vi "CreateNewFile.vi"(8 "error in (no error)":errorcluster, 11 "BenchParent in":refnum<class "BenchParent.lvclass">) -> (0 "error out":errorcluster, 2 "file path out":path, 3 "BenchParent out":refnum<class "BenchParent.lvclass">)   [LabVIEW 2024, in "BenchParent.lvclass"]
uses:
  BenchParent.lvclass
  <vilib>/numeric/Random Number (Range) DBL.vi
  BenchParent.lvclass/BenchParent.ctl
panel:
  out "Waveform Graph":waveform(dbl)(graph)
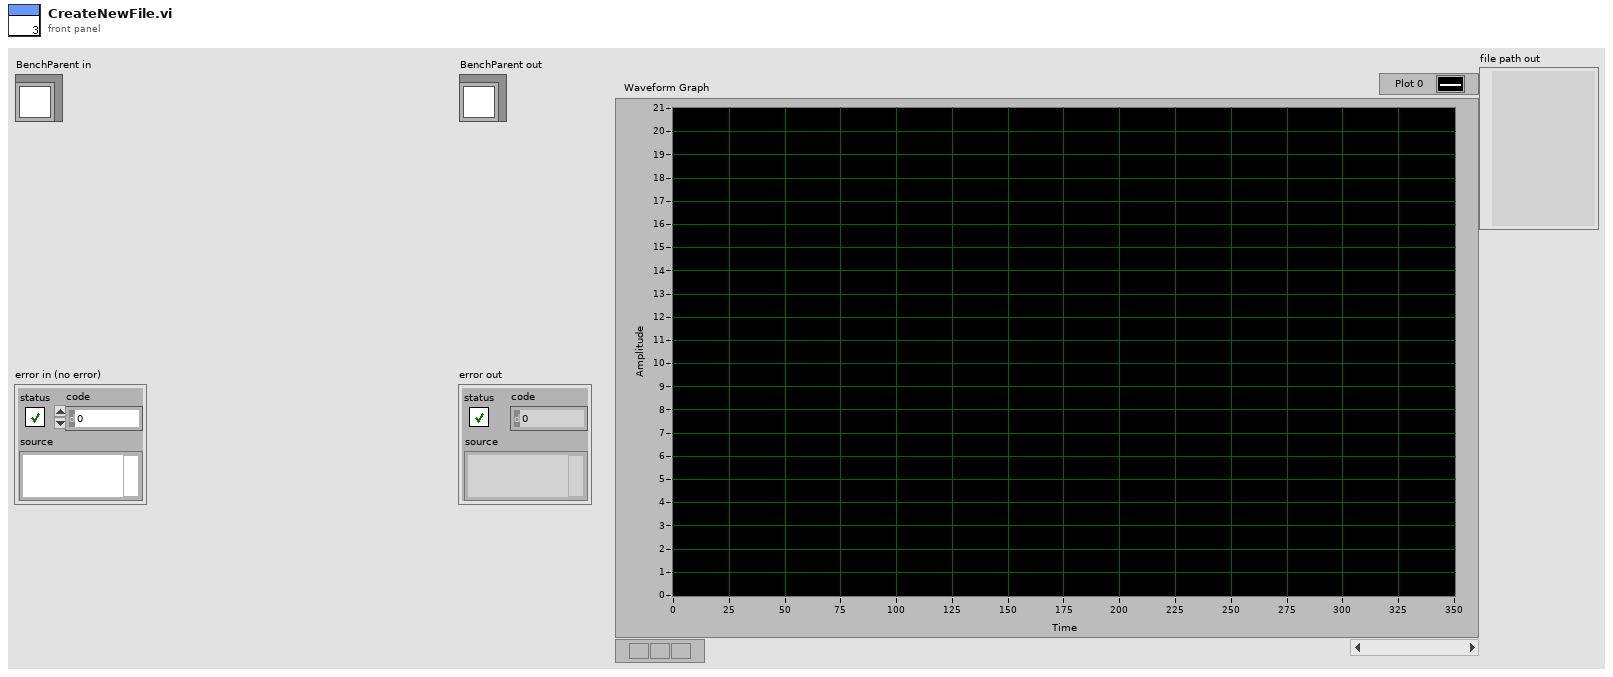
[diagram p1: front panel]
types:
  T1 = enum16{"open", "open or create", "create or replace", "create", "open (read-only)"}
  T2 = cluster{"Duration":dbl, "Level":dbl, "Noise":dbl}[]
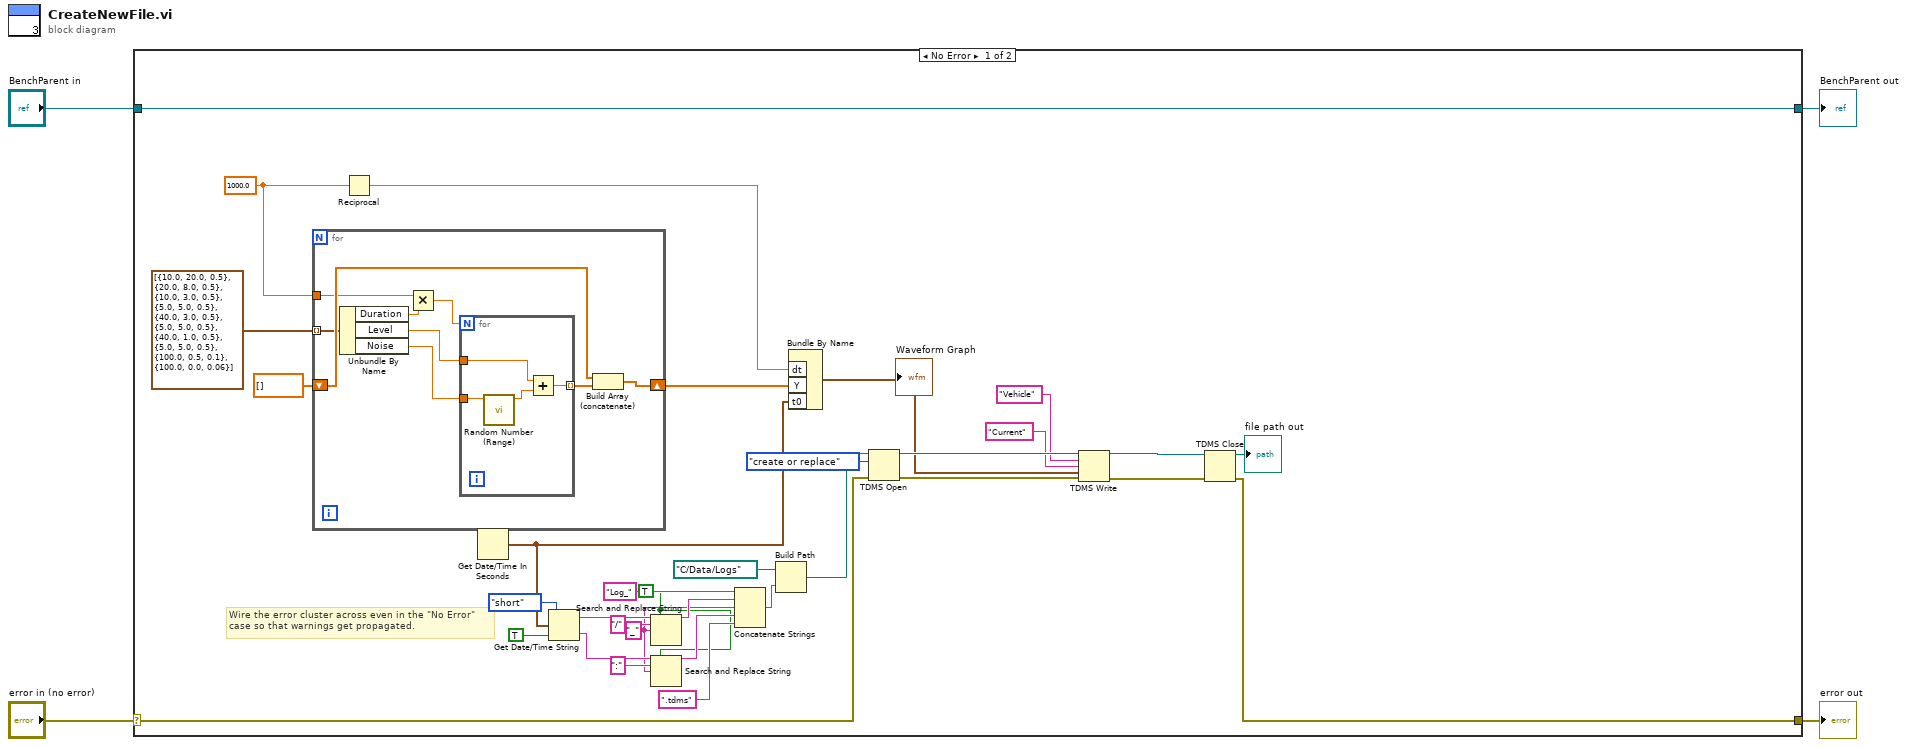
[diagram p0: block diagram]
diagram:
  n1 = case shown="No Error" "error in (no error)" {
    selector: "error in (no error)" -> [w23 w52]
    tunnel: [w24 w52] -> w3
    tunnel: [w37 w51] -> w1
    tunnel: "BenchParent in" -> [w37 w51]
    frame No Error {
      w5 = TRUE ("replace all? (F)")
      w11 = "_" ("replace string (\"\")")
      w33 = 1000.0
      # "Wire the error cluster across even in the \"No Error\"\ncase so that warnings get propagated."
      n2 = for {
        shift-right: [w44] -> w34
        shift-left: dbl[] [] -> [w43]
        tunnel: T2 [{"Duration"=10.0, "Level"=20.0, "Noise"=0.5}, {"Duration"=20.0, "Level"=8.0, "Noise"=0.5}, {"Duration"=10.0, "Level"=3.0, "Noise"=0.5}, {"Duration"=5.0, "Level"=5.0, "Noise"=0.5}, {"Duration"=40.0, "Level"=3.0, "Noise"=0.5}, {"Duration"=5.0, "Level"=5.0, "Noise"=0.5}, {"Duration"=40.0, "Level"=1.0, "Noise"=0.5}, {"Duration"=5.0, "Level"=5.0, "Noise"=0.5}, {"Duration"=100.0, "Level"=0.5, "Noise"=0.1}, {"Duration"=100.0, "Level"=0.0, "Noise"=0.06}] -> [w42] mode=indexing
        tunnel: w33 -> [w39]
        n3 = Unbundle By Name(w42) -> ("Duration"=w41:dbl, "Level"=w40:dbl, "Noise"=w38:dbl)
        n4 = Multiply(x=w39, y=w41) -> (x*y=w46:dbl)
        n5 = for {
          N: w46 -> [_]
          tunnel: w40 -> [w50]
          tunnel: [w48] -> w45 mode=indexing
          tunnel: w38 -> [w47]
          n6 = call-poly <vilib>:"Random Number (Range).vi"("upper bound (100)"=w47) -> ("number"=w49:dbl)  [unwired: 10 in]
          n7 = Add(x=w50, y=w49) -> (x+y=w48:dbl)
        }
        n8 = Build Array (concatenate)(w43, w45) -> (w44:dbl[])
      }
      n9 = Reciprocal(x=w33) -> (1/x=w32:dbl)
      n10 = Get Date/Time In Seconds() -> (seconds since 1Jan1904=w21:timestamp)
      n11 = Get Date/Time String(date format (0)=enum16{"short", "long", "abbreviated"}."short", seconds (now)=w21, want seconds? (F)=TRUE) -> (date string=w19:string, time string=w15:string)
      n12 = Search and Replace String(replace all?=w5, input string=w19, search string="/", replace string=w11) -> (result string=w16:string)  [unwired: 4 in, 3 out]
      n13 = Search and Replace String(replace all?=w5, input string=w15, search string=":", replace string=w11) -> (result string=w10:string)  [unwired: 4 in, 3 out]
      n14 = Concatenate Strings("Log_", w16, w11, w10, ".tdms" ("string")) -> (w13:string)
      n15 = Build Path(base path=path "C:/Data/Logs" ("file path"), name or relative path=w13) -> (appended path=w12:path)
      n16 = Bundle By Name("dt"=w32, "Y"=w34, "t0"=w21) -> (w30:waveform(dbl))  [unwired: 1 in]
      "Waveform Graph" <- w30
      n17 = TDMS Open(8:w23, 10:T1."create or replace" ("operation (0:open)"), 11:w12) -> (0:w25:errorcluster, 3:w31:refnum<k34>)  [unwired: 4 in]
      n18 = TDMS Write(0:w31, 5:"Vehicle" ("group name in (Untitled)"), 7:"Current" ("channel name(s) in (Untitled)"), 9:w30, 11:w25) -> (4:w27:refnum<k34>, 15:w26:errorcluster)  [unwired: 1 in, 2 out]
      n19 = TDMS Close(8:w26, 11:w27) -> (0:w24:errorcluster, 3:→"file path out":path)
    }
    frame Error {
    }
  }
  "error out" <- w3
  "BenchParent out" <- w1
